vi "View.vi"(8 "error in (no error)":errorcluster, 10 "Debugger":refnum<class "Debug Process.lvclass">, 11 "Process Tree View In":refnum<class "Process Tree View.lvclass">) -> (0 "error out":errorcluster, 3 "Process Tree View Out":refnum<class "Process Tree View.lvclass">)   [LabVIEW 2020, in "Process Tree View.lvclass"]
uses:
  Process Tree View.lvclass
  C:/Users/anton/Documents/GitHub/triarc-debugger/source/Debug View/Debug View.lvclass
  Process/Debug Process.lvclass
  Process/Debug Process.lvclass/Debug Process.ctl
  Debug View/Debug View.lvclass/Debug View.ctl
  Process Tree View.lvclass/Process Tree View.ctl
  Process Tree View Model/Process Tree View Model.lvclass
  Debug View/Debug View.lvclass
panel:
  in  "Tree Control":string(tree)
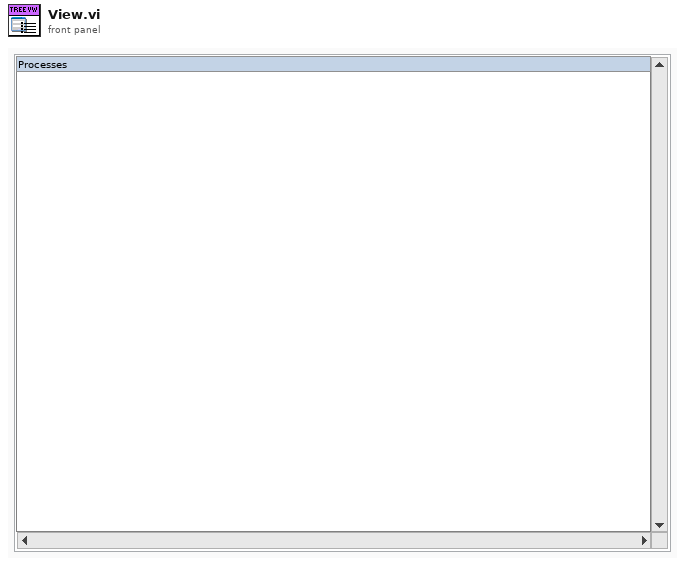
[diagram p1: front panel]
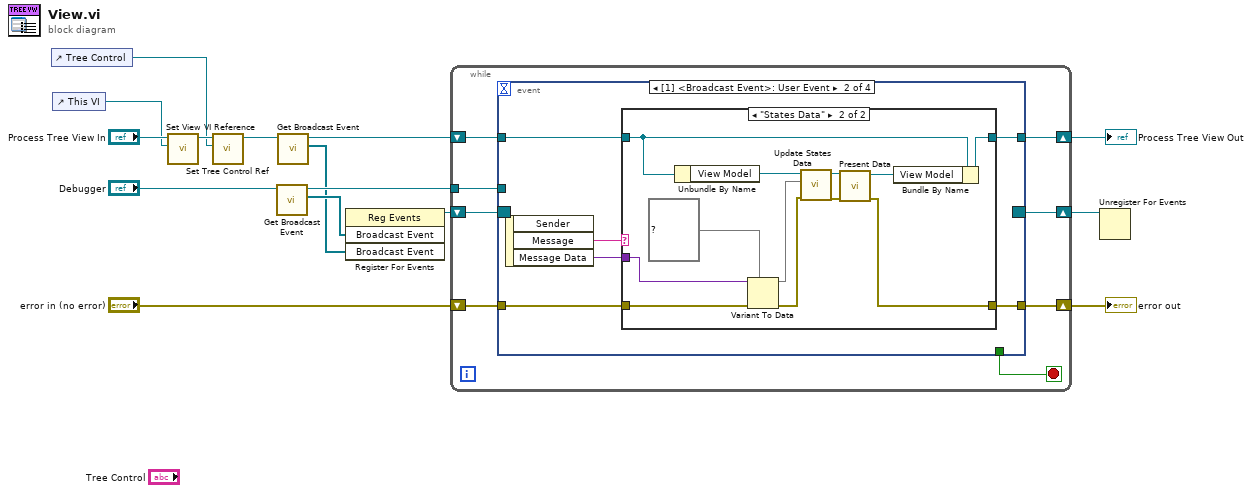
[diagram p0: block diagram]
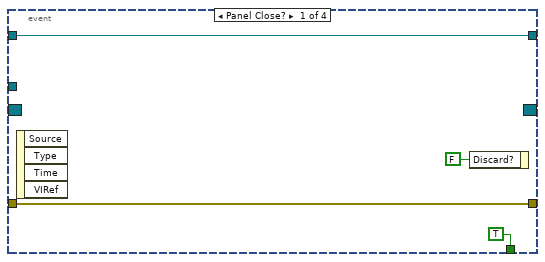
[diagram p2: hidden frame]
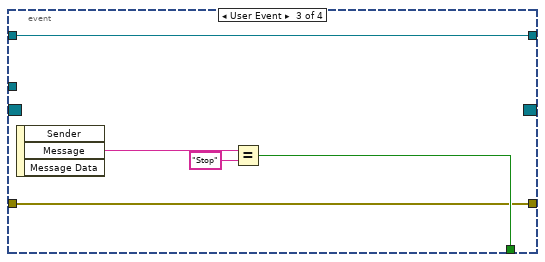
[diagram p4: hidden frame]
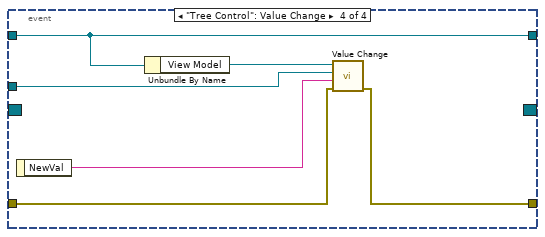
[diagram p5: hidden frame]
diagram:
  n1 = control-ref of="Tree Control"() -> (w1:refnum<vi>)
  n2 = control-ref of="This VI"() -> (w3:refnum<vi>)
  n3 = call "Set View VI Reference.vi"("View VI ref"=w3, "Debug View in"="Process Tree View In") -> ("Debug View out"=w4:refnum<class "Process Tree View.lvclass">)  [unwired: 8 in, 1 out]
  n4 = call "Set Tree Control Ref.vi"("Tree Reference"=w1, "Process Tree View in"=w4) -> ("Process Tree View out"=w2:refnum<class "Process Tree View.lvclass">)  [unwired: 8 in, 1 out]
  n5 = call "Get Broadcast Event.vi"("Process in"="Debugger") -> ("Broadcast Event"=w8:refnum<user-event>[], "Process out"=w10:refnum<class "Debug Process.lvclass">)  [unwired: 8 in, 1 out]
  n6 = call "Get Broadcast Event.vi"("Debug View In"=w2) -> ("Broadcast Event"=w5:refnum<user-event>[], "Debug View Out"=w6:refnum<class "Process Tree View.lvclass">)  [unwired: 8 in, 1 out]
  n7 = register-events(w8, w5) -> (reference out=w9:refnum<event-registration>)  [unwired: 2 in, 1 out]
  n8 = while {
    shift-right: [w22] -> w15
    shift-left: w6 -> [w23]
    shift-right: [w21] -> w14
    shift-left: "error in (no error)" -> [w20]
    shift-right: [w19] -> w12
    shift-left: w9 -> [w18]
    tunnel: w10 -> [w17]
    stop <- w16 stop-if-true
    n9 = event shown="[1] <Broadcast Event>: User Event" {
      selector: w18 -> [_ _ _ _]
      dyn-events: [_ _ _ _] -> w19
      timeout: _ -> [_ _ _ _]
      tunnel: w23 -> [w27 w29 w48 w58]
      tunnel: [w27 w28 w48 w58] -> w22
      tunnel: [w26 w32 w49 w55] -> w21
      tunnel: w20 -> [w26 w31 w49 w54]
      tunnel: w17 -> [_ _ _ w56]
      tunnel: [TRUE ("Discard?") _ w50 _] -> w16
      event Panel Close? {
        n10 = event-data() -> ()  [unwired: 1 in, 4 out]
        n11 = event-data("Discard?"=FALSE) -> ()  [unwired: 1 in, 1 out]
      }
      event User Event {
        n12 = event-data() -> ("Message"=w33:string, "Message Data"=w30:variant)  [unwired: 1 in, 1 out]
        n13 = case shown="\"States Data\"" w33 {
          tunnel: [w35 w36] -> w32
          tunnel: w31 -> [w35 w47]
          tunnel: w30 -> [_ w46]
          tunnel: w29 -> [w34 w45]
          tunnel: [w34 w43] -> w28
          frame Default {
          }
          frame "States Data" {
            n14 = Unbundle By Name(w45) -> ("View Model"=w44:refnum<class "Process Tree View Model.lvclass">)
            n15 = Variant To Data(error in=w47, type=map{string, string} {} ("State Map"), Variant=w46) -> (data=w40:map{string, string}, error out=w37:errorcluster)
            n16 = call "Update States Data.vi"("error in (no error)"=w37, "State Map"=w40, "List Seen Processes View Model In"=w44) -> ("error out"=w38:errorcluster, "List Seen Processes View Model Out"=w41:refnum<class "Process Tree View Model.lvclass">)  [unwired: 7 in]
            n17 = call "Present Data.vi"("error in (no error)"=w38, "List Seen Processes View Model In"=w41) -> ("error out"=w36:errorcluster, "List Seen Processes View Model Out"=w42:refnum<class "Process Tree View Model.lvclass">)  [unwired: 8 in]
            n18 = Bundle By Name(cluster=w45, "View Model"=w42) -> (w43:refnum<class "Process Tree View.lvclass">)
          }
        }
      }
      event User Event {
        n19 = event-data() -> ("Message"=w52:string)  [unwired: 1 in, 2 out]
        n20 = Equal?(x=w52, y="Stop") -> (x = y?=w50:bool)
      }
      event "Tree Control": Value Change {
        n21 = event-data() -> ("NewVal"=w53:string)  [unwired: 1 in]
        n22 = Unbundle By Name(w58) -> ("View Model"=w57:refnum<class "Process Tree View Model.lvclass">)
        n23 = call-dynamic "Value Change.vi"("error in (no error)"=w54, "New Value"=w53, "Debugger"=w56, "List Box View Model In"=w57) -> ("error out"=w55:errorcluster)  [unwired: 6 in, 1 out]
      }
    }
  }
  "error out" <- w14
  "Process Tree View Out" <- w15
  n24 = Unregister For Events(event registration refnum=w12) -> ()  [unwired: 1 in, 1 out]
